vi "sensor2 cal data.vi"(11 "input":waveform(dbl)[](array[waveform])) -> (3 "output":waveform(dbl)[](array[waveform]))   [LabVIEW 2013]
panel:
  in  "숫자형":u8
  out "XY 그래프":cluster{dbl[], dbl[]}(graph)
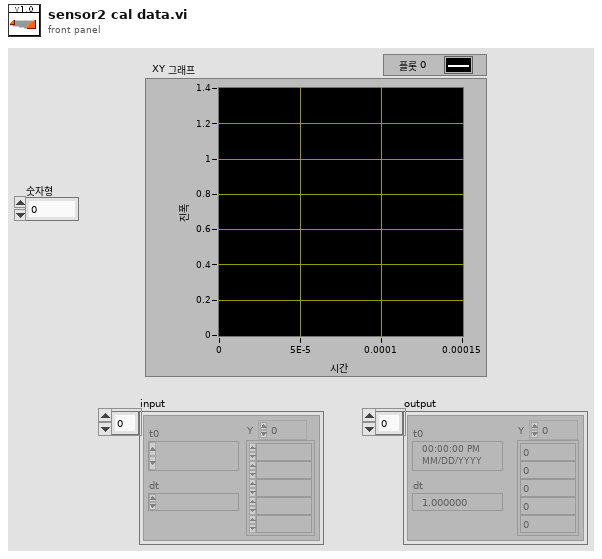
[diagram p1: front panel]
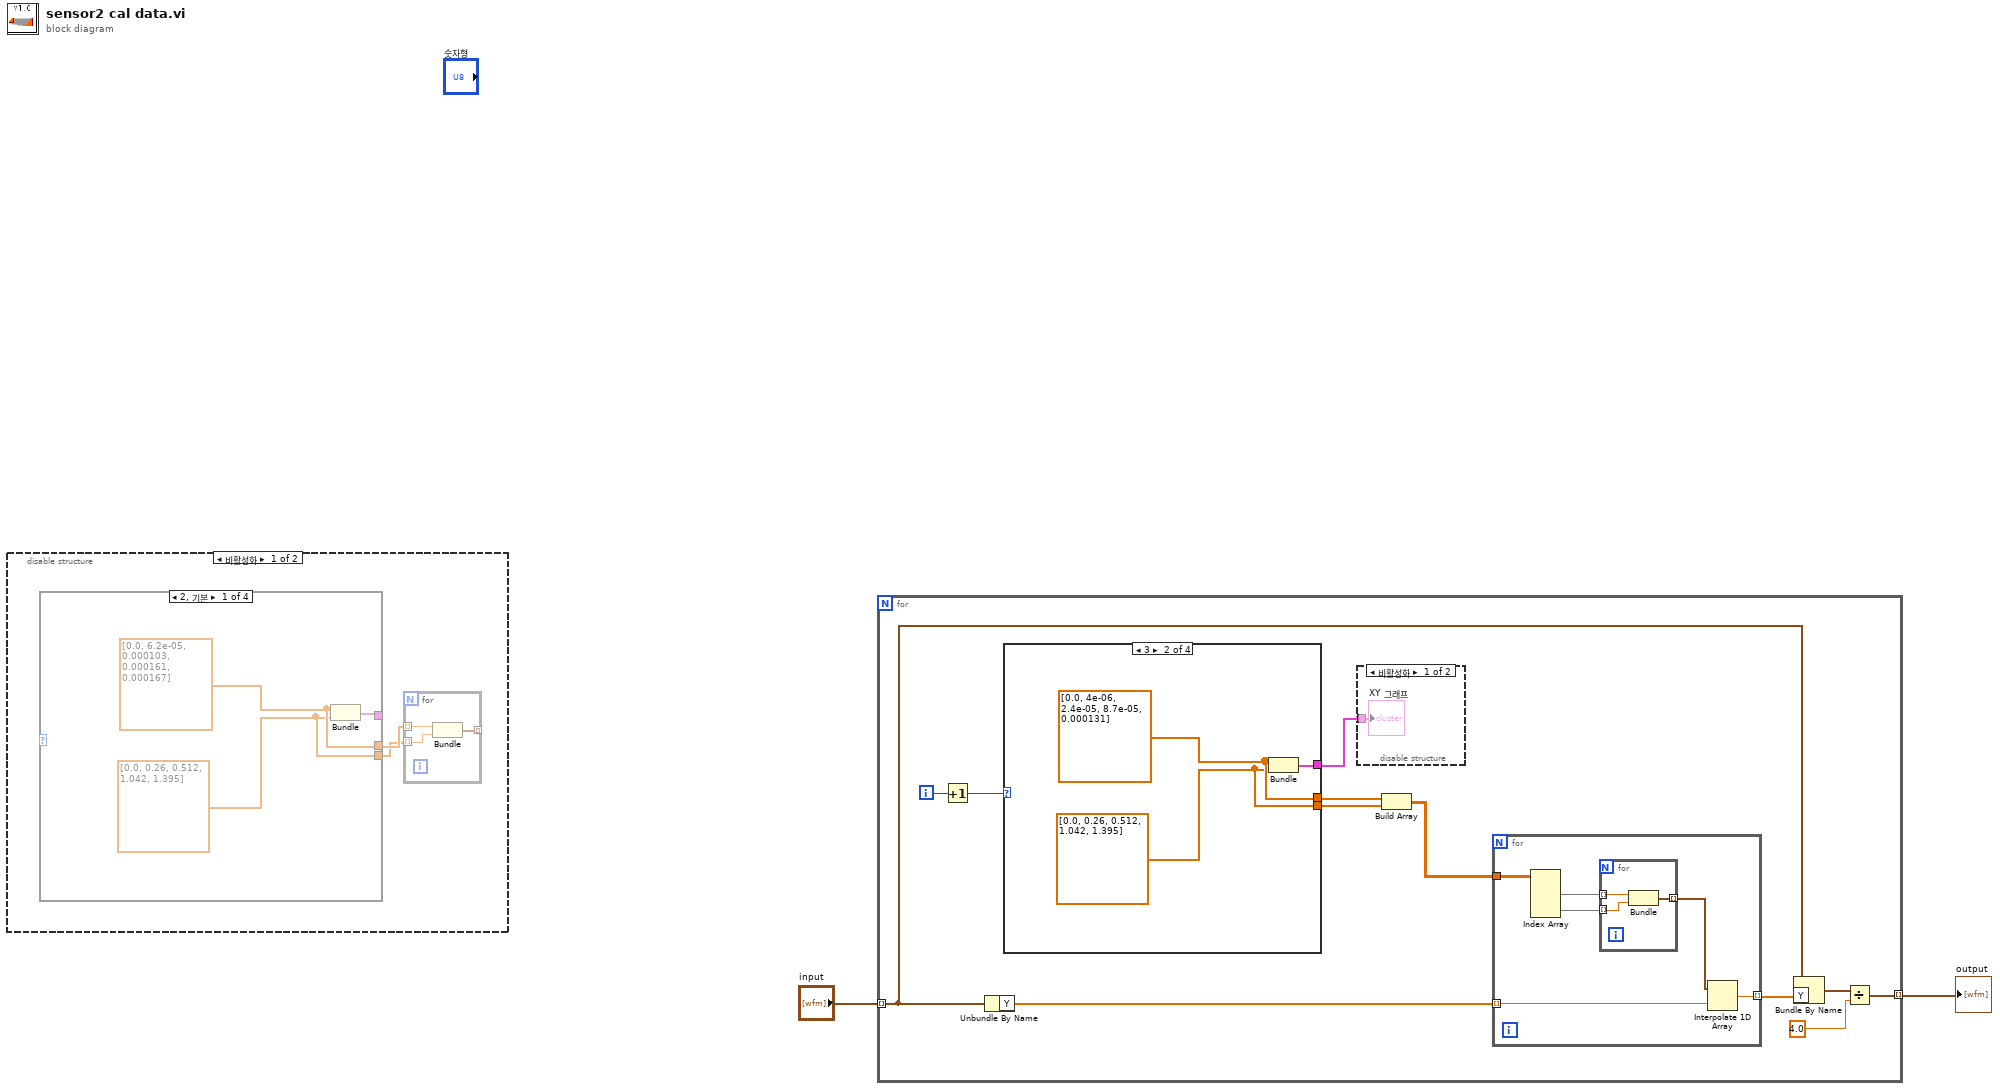
[diagram p0: block diagram]
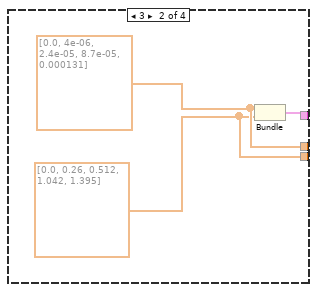
[diagram p2: hidden frame]
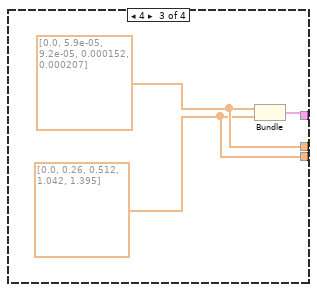
[diagram p3: hidden frame]
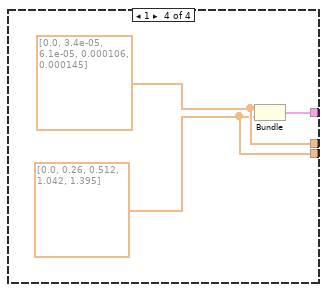
[diagram p4: hidden frame]
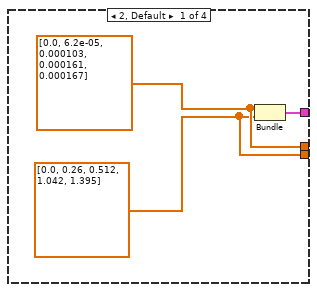
[diagram p7: hidden frame]
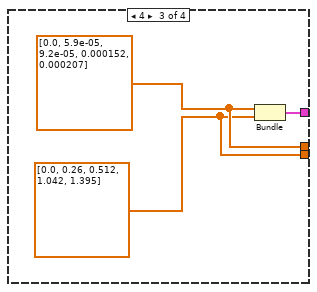
[diagram p8: hidden frame]
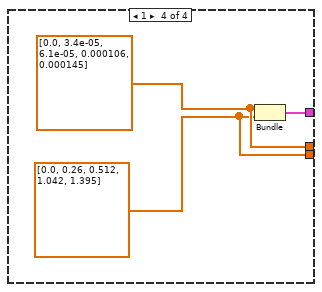
[diagram p9: hidden frame]
diagram:
  n1 = disable-structure shown="비활성화" {
    frame Disabled {
      n2 = case shown="2, 기본" {
        selector: _ -> [_ _ _ _]
        tunnel: [w10 w13 w16 w19] -> _
        tunnel: [w9 w12 w15 w18] -> w4
        tunnel: [w8 w11 w14 w17] -> w3
        frame 2, Default {
          w8 = dbl[] [0.0, 0.26, 0.512, 1.042, 1.395]
          w9 = dbl[] [0.0, 6.2e-05, 0.000103, 0.000161, 0.000167]
          n3 = Bundle(w9, w8) -> (w10:cluster{dbl[], dbl[]})  [unwired: 1 in]
        }
        frame 3 {
          w11 = dbl[] [0.0, 0.26, 0.512, 1.042, 1.395]
          w12 = dbl[] [0.0, 4e-06, 2.4e-05, 8.7e-05, 0.000131]
          n4 = Bundle(w12, w11) -> (w13:cluster{dbl[], dbl[]})  [unwired: 1 in]
        }
        frame 4 {
          w14 = dbl[] [0.0, 0.26, 0.512, 1.042, 1.395]
          w15 = dbl[] [0.0, 5.9e-05, 9.2e-05, 0.000152, 0.000207]
          n5 = Bundle(w15, w14) -> (w16:cluster{dbl[], dbl[]})  [unwired: 1 in]
        }
        frame 1 {
          w17 = dbl[] [0.0, 0.26, 0.512, 1.042, 1.395]
          w18 = dbl[] [0.0, 3.4e-05, 6.1e-05, 0.000106, 0.000145]
          n6 = Bundle(w18, w17) -> (w19:cluster{dbl[], dbl[]})  [unwired: 1 in]
        }
      }
      n7 = for {
        tunnel: w4 -> [w7] mode=indexing
        tunnel: w3 -> [w6] mode=indexing
        tunnel: [w5] -> _ mode=indexing
        n8 = Bundle(w7, w6) -> (w5:cluster{dbl, dbl})  [unwired: 1 in]
      }
    }
    frame Enabled {
    }
  }
  n9 = for {
    tunnel: "input" -> [w20] mode=indexing
    tunnel: [w24] -> w1 mode=indexing
    i -> [w22]
    n10 = Increment(x=w22) -> (x+1=w21:i32)
    n11 = Unbundle By Name(w20) -> ("Y"=w30:dbl[])
    n12 = case shown="3" w21 {
      tunnel: [w35 w38 w41 w44] -> w23
      tunnel: [w34 w37 w40 w43] -> w28
      tunnel: [w33 w36 w39 w42] -> w29
      frame 2, Default {
        w33 = dbl[] [0.0, 0.26, 0.512, 1.042, 1.395]
        w34 = dbl[] [0.0, 6.2e-05, 0.000103, 0.000161, 0.000167]
        n13 = Bundle(w34, w33) -> (w35:cluster{dbl[], dbl[]})  [unwired: 1 in]
      }
      frame 3 {
        w36 = dbl[] [0.0, 0.26, 0.512, 1.042, 1.395]
        w37 = dbl[] [0.0, 4e-06, 2.4e-05, 8.7e-05, 0.000131]
        n14 = Bundle(w37, w36) -> (w38:cluster{dbl[], dbl[]})  [unwired: 1 in]
      }
      frame 4 {
        w39 = dbl[] [0.0, 0.26, 0.512, 1.042, 1.395]
        w40 = dbl[] [0.0, 5.9e-05, 9.2e-05, 0.000152, 0.000207]
        n15 = Bundle(w40, w39) -> (w41:cluster{dbl[], dbl[]})  [unwired: 1 in]
      }
      frame 1 {
        w42 = dbl[] [0.0, 0.26, 0.512, 1.042, 1.395]
        w43 = dbl[] [0.0, 3.4e-05, 6.1e-05, 0.000106, 0.000145]
        n16 = Bundle(w43, w42) -> (w44:cluster{dbl[], dbl[]})  [unwired: 1 in]
      }
    }
    n17 = disable-structure shown="비활성화" {
      disable-tunnel: w23 -> [w32 _]
      frame Disabled {
        "XY 그래프" <- w32
      }
      frame Enabled {
      }
    }
    n18 = Build Array(w28, w29) -> (w27:dbl[][])
    n19 = for {
      tunnel: w27 -> [w46]
      tunnel: [w48] -> w31 mode=indexing
      tunnel: w30 -> [w47] mode=indexing
      n20 = Index Array(array=w46) -> (element #1=w50:dbl[], element #2=w49:dbl[])  [unwired: 4 in]
      n21 = for {
        tunnel: w50 -> [w53] mode=indexing
        tunnel: w49 -> [w52] mode=indexing
        tunnel: [w51] -> w45 mode=indexing
        n22 = Bundle(w53, w52) -> (w51:cluster{dbl, dbl})  [unwired: 1 in]
      }
      n23 = Interpolate 1D Array(1:w47, 2:w45) -> (0:w48:dbl)
    }
    n24 = Bundle By Name(cluster=w20, "Y"=w31) -> (w25:waveform(dbl))
    n25 = Divide(x=w25, y=4.0) -> (x/y=w24:waveform(dbl))
  }
  "output" <- w1
